vi "External Update.vi"(8 "error in":errorcluster, 9 "Value":variant, 10 "Parameter":string, 11 "Config in":refnum<class "Configuration.lvclass">) -> (0 "error out":errorcluster, 3 "Config out":refnum<class "Configuration.lvclass">)   [LabVIEW 2020, in "cycling structure demo UI.lvlib" / "Configuration.lvclass"]
doc: "____\nPeloton Config 2.0.0.6\nCopyright (c) 2024, Peloton"
uses:
  Configuration.lvclass
  C:/Program Files (x86)/National Instruments/LabVIEW 2020/vi.lib/Peloton/Peloton Config/DCFG Framework/Configuration_class/Configuration.lvclass
  <vilib>/Peloton/Peloton Config/DCFG Framework/Configuration_class/Configuration.lvclass/Configuration.ctl
  Configuration.lvclass/Configuration.ctl
  <vilib>/Peloton/Peloton Config/DCFG Framework/Configuration_class/Get Name.vi
  Get Configuration.vi
  Set Configuration.vi
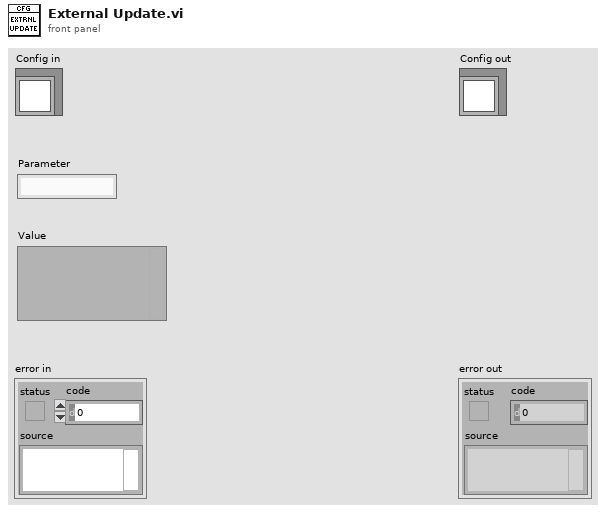
[diagram p1: front panel]
types:
  T1 = typedef "cycling structure demo UI.lvlib/Configuration.lvclass/Configuration--cluster.ctl" = cluster{"Random Path":path}
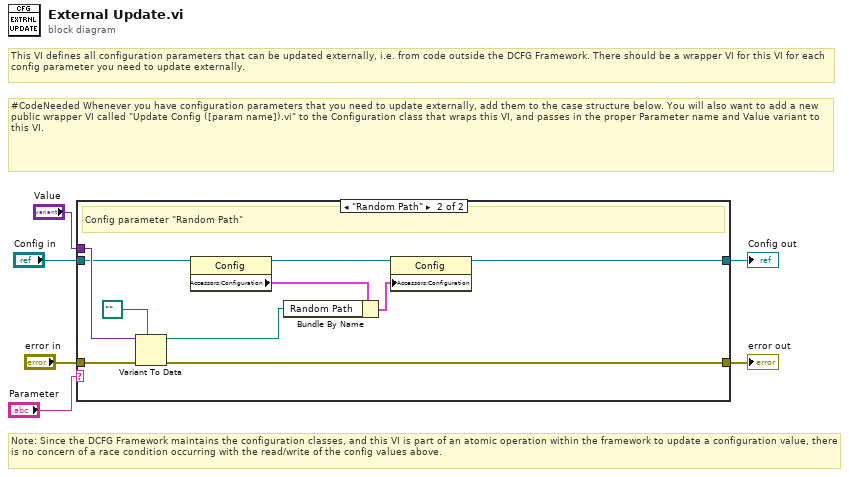
[diagram p0: block diagram]
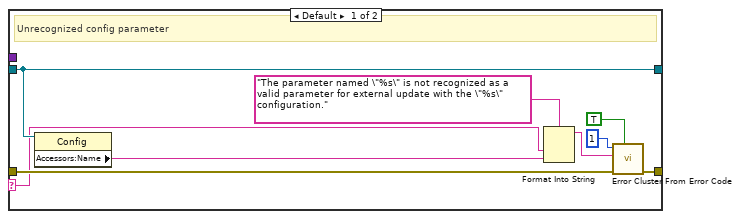
[diagram p2: hidden frame]
diagram:
  # "Note: Since the DCFG Framework maintains the configuration classes, and this VI is part of an atomic operation within the framework to update a configuration value, there is no concern of a race condition occurring with the read/write of the config values above."
  # "#CodeNeeded Whenever you have configuration parameters that you need to update externally, add them to the case structure below. You will also want to add a new public wrapper VI called \"Update Config ([param name]).vi\" to the Configuration class that wraps this VI, and passes in the proper Parameter name and Value variant to this VI."
  # "This VI defines all configuration parameters that can be updated externally, i.e. from code outside the DCFG Framework. There should be a wrapper VI for this VI for each config parameter you need to update externally."
  n1 = case shown="\"Random Path\"" "Parameter" {
    selector: "Parameter" -> [w8 _]
    tunnel: "error in" -> [w15 w25]
    tunnel: [w14 w23] -> w4
    tunnel: [w10 w18] -> w3
    tunnel: "Config in" -> [w10 w22]
    tunnel: "Value" -> [_ w24]
    frame Default {
      # "Unrecognized config parameter"
      n2 = property class="Config"(reference=w10) -> ("Accessors:Name"=w9:string)  [unwired: 1 in, 2 out]
      n3 = Format Into String(format string="The parameter named \"%s\" is not recognized as a valid parameter for external update with the \"%s\" configuration.", w8, w9) -> (resulting string=w11:string)  [unwired: 2 in, 1 out]
      n4 = call <vilib>:"Error Cluster From Error Code.vi"("show call chain? (False)"=TRUE, "error in (no error)"=w15, "error message (\"\")"=w11, "error code (0)"=1) -> ("error out"=w14:errorcluster)  [unwired: 5 in]
    }
    frame "Random Path" {
      # "Config parameter \"Random Path\""
      n5 = Variant To Data(error in=w25, type=path "" ("Random Path"), Variant=w24) -> (data=w20:path, error out=w23:errorcluster)
      n6 = property class="Config"(reference=w22) -> (reference out=w19:refnum<class "Configuration.lvclass">, "Accessors:Configuration"=w21:T1)  [unwired: 1 in, 1 out]
      n7 = Bundle By Name(cluster=w21, "Random Path"=w20) -> (w17:T1)
      n8 = property class="Config"(reference=w19, "Accessors:Configuration"=w17) -> (reference out=w18:refnum<class "Configuration.lvclass">)  [unwired: 1 in, 1 out]
    }
  }
  "error out" <- w4
  "Config out" <- w3
